vi "FromLabVIEW_Wrap.vi"(4 "TypeMap in":refnum<class "TypeMap.lvclass">, 8 "error in (no error)":errorcluster, 11 "object in":refnum<class>) -> (0 "error out":errorcluster, 2 "DbRow":variant)   [LabVIEW 2020, in "ORM.lvlib" / "TypeMap.lvclass"]
uses:
  TypeMap.lvclass
  <vilib>/Viviota/shared/ORM_lib.lvlibp/ObjectMap/ObjectMap.lvclass
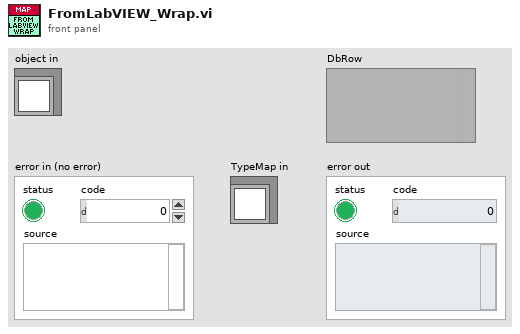
[diagram p1: front panel]
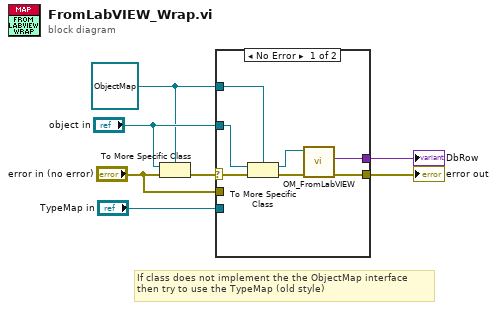
[diagram p0: block diagram]
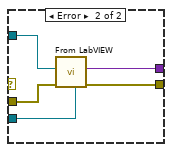
[diagram p2: hidden frame]
diagram:
  w1 = refnum<class "ObjectMap.lvclass"> refnum ("ORM_lib.lvlibp:ObjectMap")
  # "If class does not implement the the ObjectMap interface\nthen try to use the TypeMap (old style)"
  n1 = To More Specific Class(target class=w1, reference="object in", error in="error in (no error)") -> (error out=w4:errorcluster)  [unwired: 1 out]
  n2 = case shown="No Error" w4 {
    selector: w4 -> [w14 _]
    tunnel: "TypeMap in" -> [_ w19]
    tunnel: [w9 w18] -> w6
    tunnel: [w8 w17] -> w5
    tunnel: "error in (no error)" -> [_ w16]
    tunnel: "object in" -> [w12 w15]
    tunnel: w1 -> [w10 _]
    frame No Error {
      n3 = To More Specific Class(target class=w10, reference=w12, error in=w14) -> (specific class reference=w11:refnum<class "ObjectMap.lvclass">, error out=w13:errorcluster)
      n4 = call-dynamic "OM_FromLabVIEW.vi"("error in (no error)"=w13, "ObjectMap in"=w11) -> ("error out"=w8:errorcluster, "DbRow"=w9:variant)  [unwired: 7 in, 1 out]
    }
    frame Error {
      n5 = call-dynamic "From LabVIEW.vi"("TypeMap in"=w19, "error in (no error)"=w16, "Value"=w15) -> ("error out"=w17:errorcluster, "DbRow"=w18:variant)  [unwired: 7 in]
    }
  }
  "DbRow" <- w6
  "error out" <- w5
